vi "c.vi"(8 "error in (no error)":errorcluster, 11 "OK&NG":refnum<vi>) -> (0 "error out":errorcluster, 3 "OK NG out":refnum<vi>)   [LabVIEW 2013]
uses:
  controls/Data.ctl
panel:
  out "Data":T1
  # "日期"
  # "機種名稱"
  # "機種代號"
  # "商品條碼"
  # "OK"
  # "台"
  # "NG"
  # "總計"
  # "台"
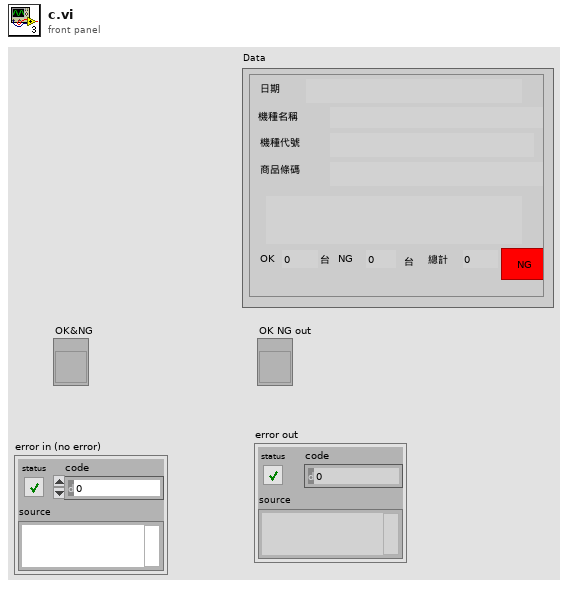
[diagram p1: front panel]
types:
  T1 = typedef "Data.ctl" = cluster{"Date":string, "BarCode1":string, "BarCode2":string, "BarCode3":string, "Message":string, "OK Count":u16, "NG Count":u16, "Total Count":u16, "ModelData":string[][], "OK&NG":bool, "COM1":refnum<visa-resource-name>, "COM2":refnum<visa-resource-name>, "IO":i32, "Time":u32}
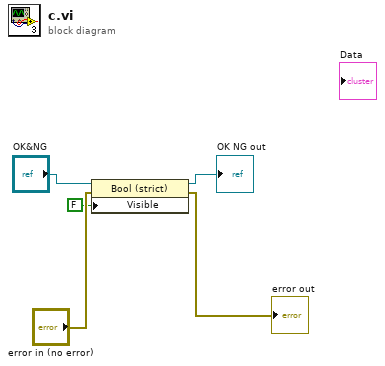
[diagram p0: block diagram]
diagram:
  n1 = property class="Bool (strict)"(reference="OK&NG", error in="error in (no error)", "Visible"=FALSE) -> (reference out=→"OK NG out":refnum<vi>, error out=→"error out":errorcluster)
